vi "deinitialize.vi"(0 "HGF_Agent":refnum<class "MoAgSy_AgentBase.lvclass">, 5 "error in (no error)":errorcluster) -> (19 "error out":errorcluster)   [LabVIEW 2009, in "MoAgSy_Base.lvlib" / "MoAgSy_AgentBase.lvclass"]
doc: "This is a dynamic dispatch VI. It can be overwritten by childclasses to release allocated recources."
uses:
  MoAgSy_AgentBase.lvclass
  HGF_BaseClasses/HGF_Visitable/HGF_Visitable.lvclass
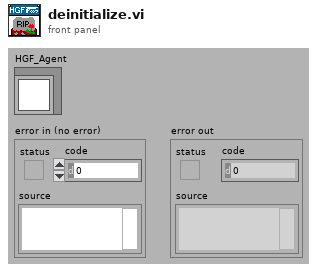
[diagram p1: front panel]
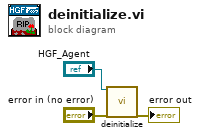
[diagram p0: block diagram]
diagram:
  n1 = call-parent "deinitialize.vi"("HGF_Factory"="HGF_Agent", "error in (no error)"="error in (no error)") -> ("error out"=→"error out":errorcluster)  [unwired: 17 in]
